vi "Status.vi"() -> ()   [LabVIEW 2018]
panel:
  in  "Exit":dbl(slide) scale=0.0..10.0
  in  "Targets":dbl(knob) scale=0.0..4.0
  out "Main PIG/IG":dbl(knob) scale=1e-07..1000.0
  in  "stop":bool
  out "LoadLock":dbl(knob) scale=1e-06..760.0
  # "mT"
  # "mT"
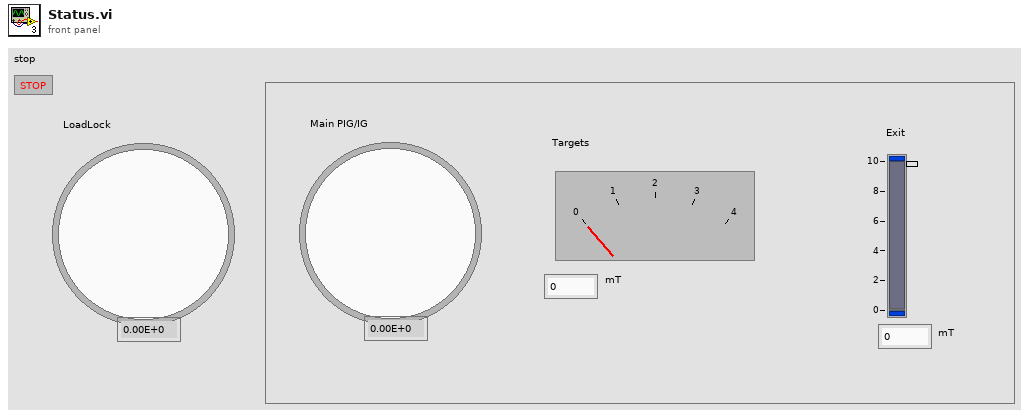
[diagram p1: front panel]
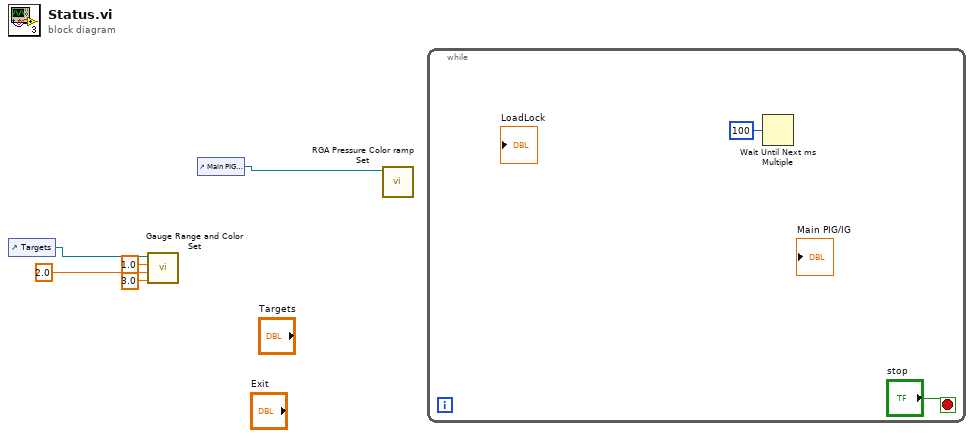
[diagram p0: block diagram]
diagram:
  n1 = control-ref of="Targets"() -> (w4:refnum<vi>)
  n2 = call "Gauge Range and Color Set.vi"("Alarm Maximum"=3.0, "Nominal Target"=2.0, "Alarm Minimum"=1.0, "reference"=w4) -> ()  [unwired: 8 in]
  n3 = control-ref of="Main PIG/IG"() -> (w5:refnum<vi>)
  n4 = call "RGA Pressure Color ramp Set.vi"("reference"=w5) -> ()  [unwired: 9 in, 2 out]
  n5 = while {
    stop <- "stop" stop-if-true
    n6 = Wait Until Next ms Multiple(millisecond multiple=u32 100) -> ()  [unwired: 1 out]
  }
